vi "Seg2Ang.vi"(9 "Distances":dbl[](array[numeric]), 10 "Segments":dbl[](array[numeric])) -> (2 "Y":dbl[](array[numeric]), 3 "X":dbl[](array[numeric]))   [LabVIEW 2012]
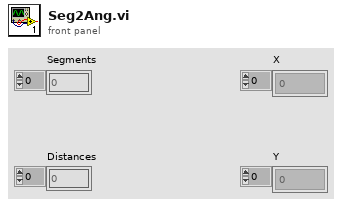
[diagram p1: front panel]
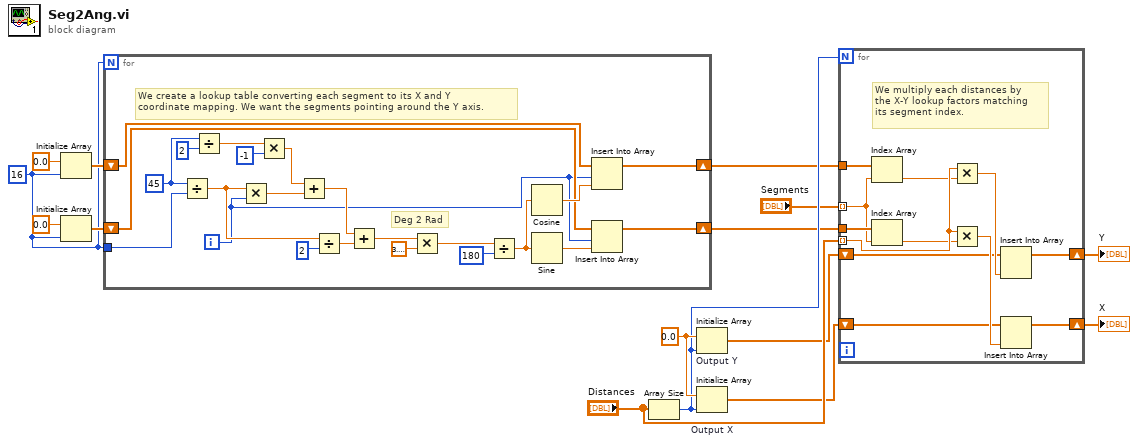
[diagram p0: block diagram]
diagram:
  w10 = 0.0 ("element")
  w11 = 16 ("dimension size")
  n1 = Initialize Array(0.0 ("element"), w11) -> (w14:dbl[])
  n2 = Initialize Array(0.0 ("element"), w11) -> (w13:dbl[])
  n3 = for {
    N: w11 -> [_]
    tunnel: w11 -> [w16]
    shift-right: [w37] -> w8
    shift-left: w14 -> [w38]
    shift-right: [w34] -> w7
    shift-left: w13 -> [w35]
    i -> [w17]
    w24 = 45
    # "We create a lookup table converting each segment to its X and Y\ncoordinate mapping. We want the segments pointing around the Y axis."
    # "Deg 2 Rad"
    n4 = Divide(x=w24, y=w16) -> (x/y=w28:dbl)
    n5 = Divide(x=w24, y=2) -> (x/y=w21:dbl)
    n6 = Multiply(x=w28, y=w17) -> (x*y=w23:dbl)
    n7 = Multiply(x=w21, y=-1) -> (x*y=w22:dbl)
    n8 = Add(x=w22, y=w23) -> (x+y=w25:dbl)
    n9 = Divide(x=w28, y=2) -> (x/y=w26:dbl)
    n10 = Add(x=w25, y=w26) -> (x+y=w18:dbl)
    n11 = Multiply(x=w18, y=3.141592653589793) -> (x*y=w31:dbl)
    n12 = Divide(x=w31, y=180) -> (x/y=w30:dbl)
    n13 = Cosine(x=w30) -> (cos(x)=w36:dbl)
    n14 = Sine(x=w30) -> (sin(x)=w33:dbl)
    n15 = Insert Into Array(array=w38, index=w17, new element=w36) -> (w37:dbl[])
    n16 = Insert Into Array(array=w35, index=w17, new element=w33) -> (w34:dbl[])
  }
  n17 = Array Size(array="Distances") -> (size(s)=w9:i32)
  n18 = Initialize Array "Output Y"(w10, w9) -> (w4:dbl[])
  n19 = Initialize Array "Output X"(w10, w9) -> (w3:dbl[])
  n20 = for {
    N: w9 -> [_]
    tunnel: w8 -> [w50]
    tunnel: w7 -> [w49]
    tunnel: "Segments" -> [w39] mode=indexing
    tunnel: "Distances" -> [w48] mode=indexing
    shift-right: [w41] -> w2
    shift-left: w4 -> [w43]
    shift-right: [w40] -> w1
    shift-left: w3 -> [w42]
    # "We multiply each distances by\nthe X-Y lookup factors matching\nits segment index."
    n21 = Index Array "Index Array"(array=w50, index=w39) -> (element=w46:dbl)
    n22 = Index Array "Index Array"(array=w49, index=w39) -> (element=w47:dbl)
    n23 = Multiply(x=w48, y=w46) -> (x*y=w45:dbl)
    n24 = Multiply(x=w48, y=w47) -> (x*y=w44:dbl)
    n25 = Insert Into Array(array=w43, new element=w45) -> (w41:dbl[])  [unwired: 1 in]
    n26 = Insert Into Array(array=w42, new element=w44) -> (w40:dbl[])  [unwired: 1 in]
  }
  "X" <- w1
  "Y" <- w2
